vi "test_exec.vi"() -> ()   [LabVIEW 2018]
doc: "MeasGUI - Measurement Graphics User Interface\nCopyright (c) 2018 Frans Korhonen\n\nMeasGUI was originally developed at Institute for Atmospheric \nand Earth System Research / Physics, Faculty of Science, \nUniversity of Helsinki, Finland\n\nAssistance, experience and feedback from following persons have been \ncritical in development of MeasGUI: Michel Attoui, Juha Kangasluoma, \nLauri Ahonen, Ella Häkkinen, Markku Kulmala and Tuukka Petäjä.\n\nThis file is part of MeasGUI.\n\nThis Source Code Form is subject to the terms of the Mozilla Public\nLicense, v. 2.0. If a copy of the MPL was not distributed with this\nfile, You can obtain one at http://mozilla.org/MPL/2.0/."
panel:
  out "standard output":string
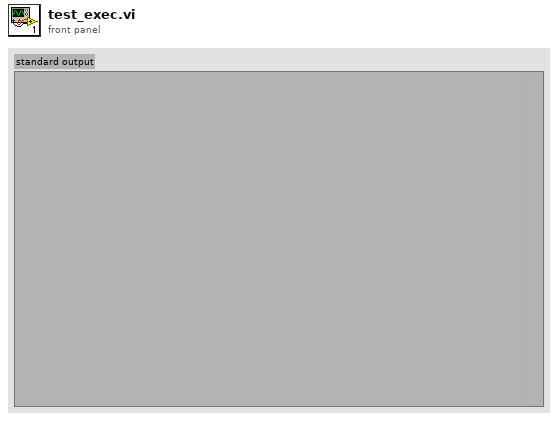
[diagram p1: front panel]
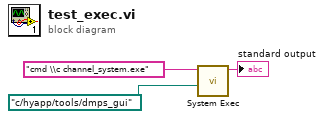
[diagram p0: block diagram]
diagram:
  n1 = call <vilib>:"System Exec.vi"("working directory"=path "c:/hyapp/tools/dmps_gui", "command line"="cmd \\c channel_system.exe") -> ("standard output"=→"standard output":string)  [unwired: 6 in, 3 out]
